vi "Stop.vi"(8 "error in":errorcluster, 11 "Scope Base in":refnum<class "Scope Base.lvclass">) -> (0 "error out":errorcluster, 3 "Scope Base out":refnum<class "Scope Base.lvclass">)   [LabVIEW 2023, in "Scope Base.lvlib" / "Scope Base.lvclass"]
uses:
  Scope Base.lvclass
  Scope Base.lvclass/Scope Base.ctl
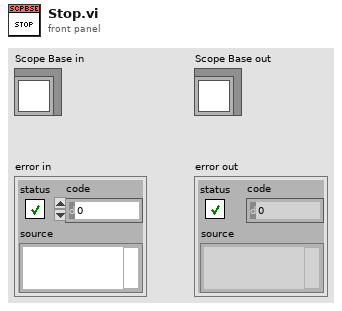
[diagram p1: front panel]
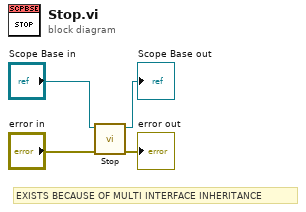
[diagram p0: block diagram]
diagram:
  # "EXISTS BECAUSE OF MULTI INTERFACE INHERITANCE"
  n1 = call-dynamic "Stop.vi"("error in"="error in", "Scope Base in"="Scope Base in") -> ("error out"=→"error out":errorcluster, "Scope Base out"=→"Scope Base out":refnum<class "Scope Base.lvclass">)  [unwired: 8 in]
